vi "DH Type to Task Type.vi"(10 "DH Type":string) -> (2 "Task Type":string)   [LabVIEW 2020, in "VolatusData.lvlib" / "DataHandlerTask.lvclass"]
uses:
  DataHandlerTask.lvclass
  DataHandlerTask.lvclass/DataHandlerTask.ctl
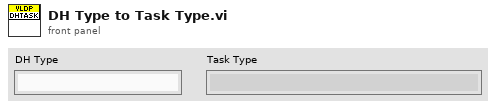
[diagram p1: front panel]
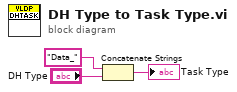
[diagram p0: block diagram]
diagram:
  n1 = Concatenate Strings("Data_", "DH Type") -> (→"Task Type":string)
